vi "Debug Write Error Cluster.vi"(4 "log no error? (T)":bool=TRUE, 5 "status and code only? (T)":bool=TRUE, 6 "include timestamp? (F)":bool, 7 "prefix (\"\")":string, 8 "error in":errorcluster, 9 "clear before next write (F)":bool, 10 "clear error after logging? (T)":bool=TRUE) -> (0 "error out":errorcluster)   [LabVIEW 2020, in "Debug Log.lvlib"]
doc: "Use this VI to log error clusters generated at various points in your program. Each time you call it, it appends <b>prefix</b> + <b>error in</b> to the displayed string, optionally including a timestamp. This VI opens on first call and remains open even after the program terminates.\n\nUse this VI in combination with <b>Debug Log:Debug Write</b> VI to log other data types."
uses:
  <vilib>/Utility/Debug Log/Debug Log.lvlib
  <vilib>/Utility/error.llb/DialogType.ctl
panel:
  in  "Warning":string="Warning"
  in  "Error":string="Error"
  in  "No Error":string="No Error"
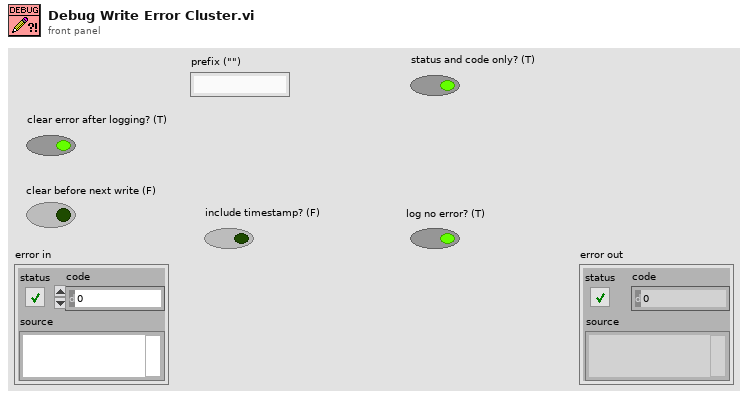
[diagram p1: front panel]
types:
  T1 = typedef "DialogType.ctl" = u16
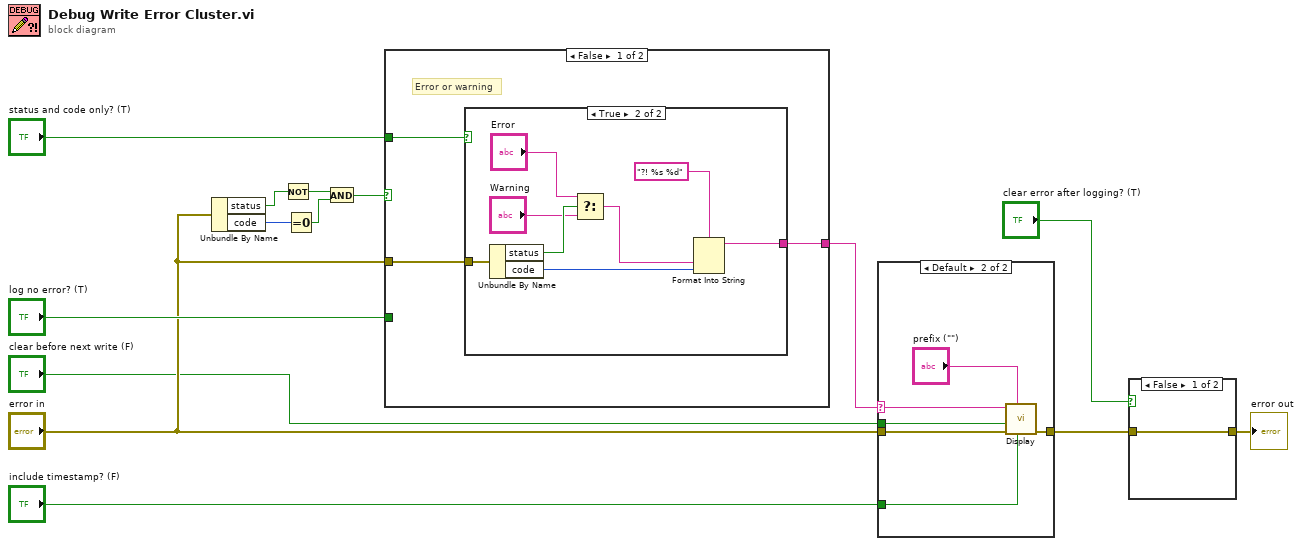
[diagram p0: block diagram]
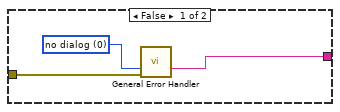
[diagram p4: hidden frame]
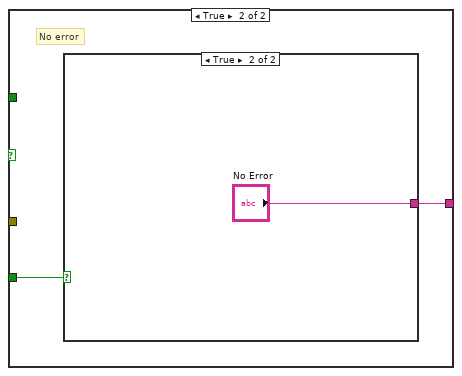
[diagram p5: hidden frame]
diagram:
  n1 = Unbundle By Name("error in") -> ("status"=w10:bool, "code"=w12:i32)
  n2 = Not(x=w10) -> (.not. x?=w9:bool)
  n3 = Equal To 0?(x=w12) -> (x = 0?=w11:bool)
  n4 = And(x=w9, y=w11) -> (x .and. y?=w8:bool)
  n5 = case shown="False" w8 {
    tunnel: "status and code only? (T)" -> [w17 _]
    tunnel: "log no error? (T)" -> [_ w30]
    tunnel: [w15 w29] -> w6
    tunnel: "error in" -> [w16 _]
    frame False {
      # "Error or warning"
      n6 = case shown="True" w17 {
        tunnel: w16 -> [w20 w28]
        tunnel: [w18 w21] -> w15
        frame False {
          w19 = T1 0 items=["no dialog", "OK message", "continue or stop message", "OK message + warnings", "continue/stop + warnings"] ("type of dialog (OK msg:1)")
          n7 = call <vilib>:"General Error Handler.vi"("type of dialog (OK msg:1)"=w19, "error in (no error)"=w20) -> ("message"=w18:string)  [unwired: 9 in, 4 out]
        }
        frame True {
          n8 = Unbundle By Name(w28) -> ("status"=w25:bool, "code"=w26:i32)
          n9 = Select(t="Error", s=w25, f="Warning") -> (s? t:f=w22:string)
          n10 = Format Into String(format string="?! %s %d", w22, w26) -> (resulting string=w21:string)  [unwired: 2 in, 1 out]
        }
      }
    }
    frame True {
      # "No error"
      n11 = case shown="True" w30 {
        tunnel: [_ "No Error"] -> w29
        frame False {
        }
        frame True {
        }
      }
    }
  }
  n12 = case shown="Default" w6 {
    selector: w6 -> [_ w34]
    tunnel: "include timestamp? (F)" -> [_ w37]
    tunnel: [w32 w36] -> w2
    tunnel: "error in" -> [w32 w35]
    tunnel: "clear before next write (F)" -> [_ w33]
    frame "" {
    }
    frame Default {
      n13 = call <vilib>:"Display.vi"("include timestamp? (F)"=w37, "prefix (\"\")"="prefix (\"\")", "error in (no error)"=w35, "clear before next write (F)"=w33, "log text"=w34) -> ("error out"=w36:errorcluster)  [unwired: 6 in]
    }
  }
  n14 = case shown="False" "clear error after logging? (T)" {
    tunnel: [w39 _] -> w3
    tunnel: w2 -> [w39 _]
    frame False {
    }
    frame True {
    }
  }
  "error out" <- w3
